vi "Unregister Event.vi"(7 "Event":refnum<class "Event.lvclass">, 8 "error in (no error)":errorcluster, 11 "View Actor in":refnum<class "View Actor.lvclass">) -> (0 "error out":errorcluster, 3 "View Actor out":refnum<class "View Actor.lvclass">)   [LabVIEW 2023, in "Event Actors.lvlib" / "View Actor.lvclass"]
doc: "Unregisters an event to the Controller by specifiying the concrete event."
uses:
  View Actor.lvclass
  View Actor.lvclass/View Actor.ctl
  Controller Actor Messages/Unregister by Name Msg/Unregister by Name Msg.lvclass
  Event/Event.lvclass
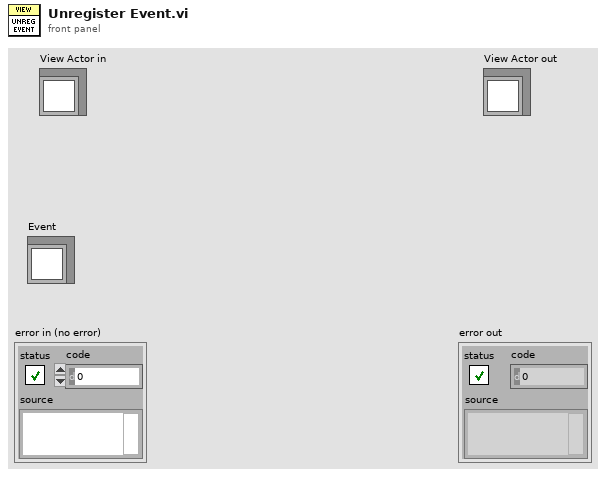
[diagram p1: front panel]
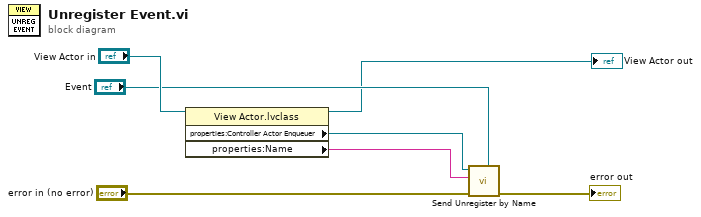
[diagram p0: block diagram]
diagram:
  n1 = property class="View Actor.lvclass"(reference="View Actor in") -> (reference out=→"View Actor out":refnum<class "View Actor.lvclass">, "properties:Controller Actor Enqueuer"=w2:refnum<class "Message Enqueuer.lvclass">, "properties:Name"=w3:string)  [unwired: 1 in, 1 out]
  n2 = call "Send Unregister by Name.vi"("Event"="Event", "error in (no error)"="error in (no error)", "View Name"=w3, "Message Enqueuer in"=w2) -> ("error out"=→"error out":errorcluster)  [unwired: 6 in, 1 out]
